vi "EditAnything.vi"(11 "Template Name":path) -> ()   [LabVIEW 2019]
uses:
  <userlib>/MicroPython/VIs/ColorText/Code.xctl
panel:
  in  "VISA resource name":refnum<visa-resource-name>
  in  "Open":bool
  in  "Save Button":bool
  in  "Code":string(xcontrol)
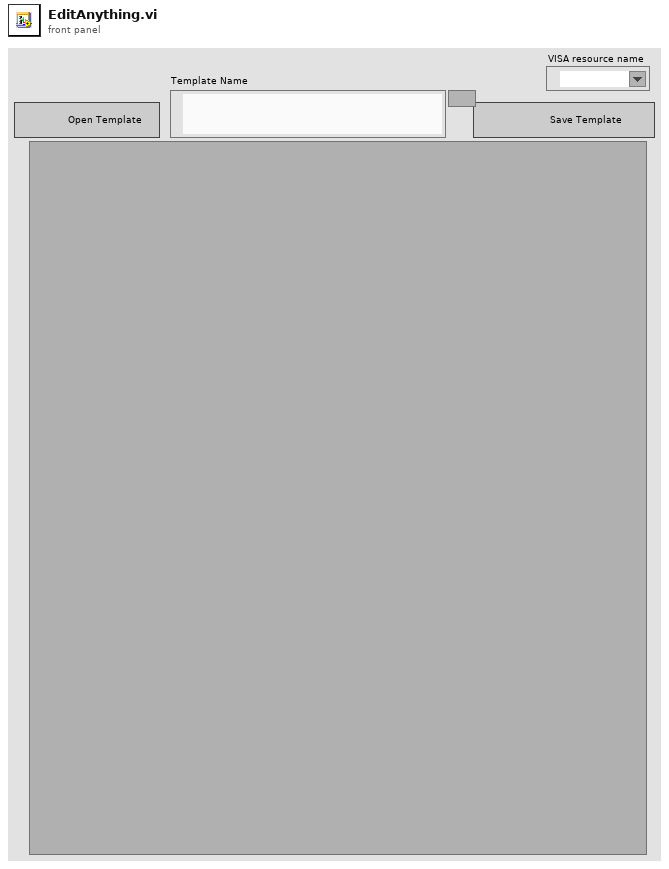
[diagram p1: front panel]
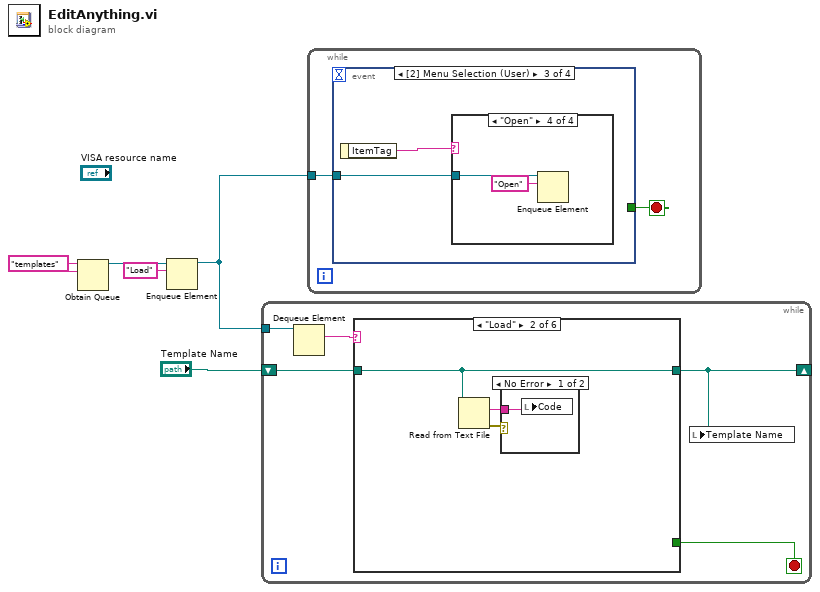
[diagram p0: block diagram]
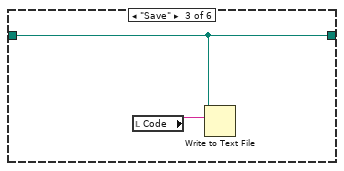
[diagram p4: hidden frame]
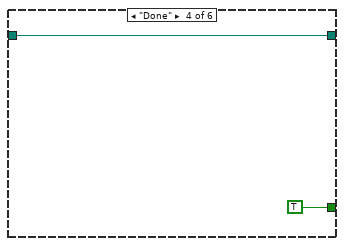
[diagram p5: hidden frame]
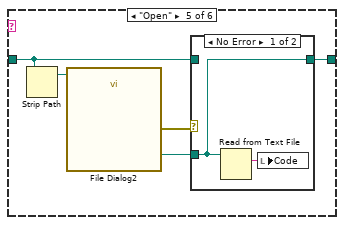
[diagram p6: hidden frame]
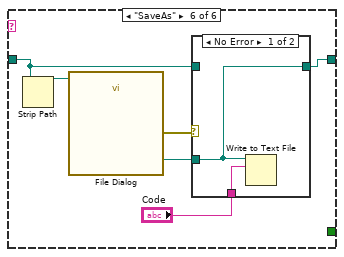
[diagram p8: hidden frame]
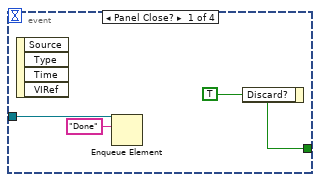
[diagram p10: hidden frame]
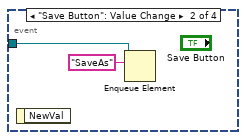
[diagram p11: hidden frame]
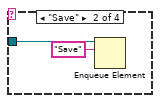
[diagram p13: hidden frame]
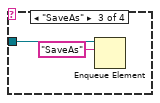
[diagram p14: hidden frame]
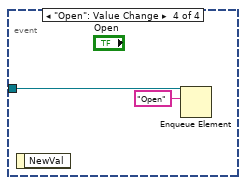
[diagram p15: hidden frame]
diagram:
  w3 = "templates" ("name (unnamed)")
  n1 = Obtain Queue(name (unnamed)=w3, element data type=w3) -> (queue out=w4:refnum<queue>)  [unwired: 3 in, 2 out]
  n2 = Enqueue Element(queue=w4, element="Load") -> (queue out=w2:refnum<queue>)  [unwired: 2 in, 2 out]
  n3 = while {
    shift-right: [w6] -> _
    shift-left: "Template Name" -> [w9]
    tunnel: w2 -> [w8]
    stop <- w7 stop-if-true
    n4 = Dequeue Element(queue=w8) -> (element=w10:string)  [unwired: 2 in, 3 out]
    n5 = case shown="\"Load\"" w10 {
      tunnel: [w11 w12 w16 w19 w20 w29] -> w6
      tunnel: w9 -> [w11 w12 w16 w19 w21 w28]
      tunnel: [_ _ _ TRUE _ _] -> w7
      frame Default {
      }
      frame "Load" {
        n6 = Read from Text File(file (use dialog)=w12) -> (text=w13:string, error out=w14:errorcluster)  [unwired: 3 in, 2 out]
        n7 = case shown="No Error" w14 {
          tunnel: w13 -> [w15 _]
          frame No Error {
            n8 = local write "Code"(w15) -> ()
          }
          frame Error {
          }
        }
      }
      frame "Save" {
        n9 = local read "Code"() -> (w17:string)
        n10 = Write to Text File(file (use dialog)=w16, text=w17) -> ()  [unwired: 2 in, 3 out]
      }
      frame "Done" {
      }
      frame "Open" {
        n11 = Strip Path(path=w21) -> (stripped path=w23:path)  [unwired: 1 out]
        n12 = call "File Dialog2"("start path"=w23) -> ("selected path"=w22:path, "error out"=w24:errorcluster)  [unwired: 11 in, 2 out]
        n13 = case shown="No Error" w24 {
          tunnel: w22 -> [w25 _]
          tunnel: [w25 w27] -> w20
          tunnel: w21 -> [_ w27]
          frame No Error {
            n14 = Read from Text File(file (use dialog)=w25) -> (text=w26:string)  [unwired: 3 in, 3 out]
            n15 = local write "Code"(w26) -> ()
          }
          frame Error {
          }
        }
      }
      frame "SaveAs" {
        n16 = Strip Path(path=w28) -> (stripped path=w32:path)  [unwired: 1 out]
        n17 = call "File Dialog"("start path"=w32) -> ("selected path"=w30:path, "error out"=w33:errorcluster)  [unwired: 11 in, 2 out]
        n18 = case shown="No Error" w33 {
          tunnel: w30 -> [w34 _]
          tunnel: "Code" -> [w35 _]
          tunnel: [w34 w36] -> w29
          tunnel: w28 -> [_ w36]
          frame No Error {
            n19 = Write to Text File(file (use dialog)=w34, text=w35) -> ()  [unwired: 2 in, 3 out]
          }
          frame Error {
          }
        }
      }
    }
    n20 = local write "Template Name"(w6) -> ()
  }
  n21 = while {
    tunnel: w2 -> [w37]
    stop <- w38 stop-if-true
    n22 = event shown="[2] Menu Selection (User)" {
      selector: _ -> [_ _ _ _]
      dyn-events: _ -> [_ _ _ _]
      timeout: _ -> [_ _ _ _]
      tunnel: [w41 _ _ _] -> w38
      tunnel: w37 -> [w39 w42 w44 w53]
      event Panel Close? {
        w41 = TRUE ("Discard?")
        n23 = event-data() -> ()  [unwired: 1 in, 4 out]
        n24 = Enqueue Element(queue=w39, element="Done") -> ()  [unwired: 2 in, 3 out]
        n25 = event-data("Discard?"=w41) -> ()  [unwired: 1 in, 1 out]
      }
      event "Save Button": Value Change {
        n26 = event-data() -> ()  [unwired: 1 in, 1 out]
        n27 = Enqueue Element(queue=w42, element="SaveAs") -> ()  [unwired: 2 in, 3 out]
      }
      event Menu Selection (User) {
        n28 = event-data() -> ("ItemTag"=w45:string)  [unwired: 1 in]
        n29 = case shown="\"Open\"" w45 {
          tunnel: w44 -> [_ w46 w48 w50]
          frame Default {
          }
          frame "Save" {
            n30 = Enqueue Element(queue=w46, element="Save") -> ()  [unwired: 2 in, 3 out]
          }
          frame "SaveAs" {
            n31 = Enqueue Element(queue=w48, element="SaveAs") -> ()  [unwired: 2 in, 3 out]
          }
          frame "Open" {
            n32 = Enqueue Element(queue=w50, element="Open") -> ()  [unwired: 2 in, 3 out]
          }
        }
      }
      event "Open": Value Change {
        n33 = event-data() -> ()  [unwired: 1 in, 1 out]
        n34 = Enqueue Element(queue=w53, element="Open") -> ()  [unwired: 2 in, 3 out]
      }
    }
  }
